vi "ASIA Pump Handler.vi"() -> ()   [LabVIEW 2021, in "Support Library.lvlib"]
uses:
  Support Library.lvlib
  ASIA Pump/Pump Settings.ctl
  <vilib>/addons/_JKI.lib/Serialization/JSON/JKI JSON Serialization.lvlib
  ASIA Pump.lvlib
panel:
  in  "stop":bool
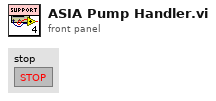
[diagram p1: front panel]
types:
  T1 = typedef "ASIA Pump.lvlib/Pump Settings.ctl" = cluster{"ASIA Pump #":i32, "channel":i32, "Simulated":bool}
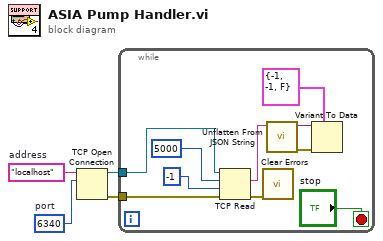
[diagram p0: block diagram]
diagram:
  w4 = u16 6340  # port
  w3 = "localhost"  # address
  n1 = TCP Open Connection(address=w3, remote port or service name=w4) -> (connection ID=w1:refnum<k5>, error out=w2:errorcluster)  [unwired: 3 in]
  n2 = while {
    tunnel: w2 -> [w7]
    tunnel: w1 -> [w6]
    stop <- "stop" stop-if-true
    n3 = TCP Read(connection ID=w6, bytes to read=5000, error in (no error)=w7, 9:-1 ("timeout ms (25000)")) -> (data out=w9:string, error out=w10:errorcluster)  [unwired: 1 in, 1 out]
    n4 = call <vilib>:"Clear Errors.vi"("error in (no error)"=w10) -> ()  [unwired: 5 in, 2 out]
    n5 = call <vilib>:"Unflatten From JSON String.vi"("JSON String"=w9) -> ("error out"=w13:errorcluster, "Variant"=w14:variant)  [unwired: 9 in]
    n6 = Variant To Data(error in=w13, type=T1 {"ASIA Pump #"=-1, "channel"=-1, "Simulated"=FALSE} ("ASIA Pump C"), Variant=w14) -> ()  [unwired: 2 out]
  }
